vi "Global 1.vi"() -> ()   [LabVIEW 2016]
panel:
  out "Yaw":dbl
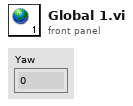
[diagram p1: front panel]
diagram:
